vi "initialize Session Data.vi"(0 "Session in":refnum<class "Remote Connection Session.lvclass">, 11 "error in":errorcluster) -> (4 "Session out":refnum<class "Remote Connection Session.lvclass">, 15 "error out":errorcluster)   [LabVIEW 2012, in "REx.lvlib" / "Remote Connection Session.lvclass"]
uses:
  Remote Connection Session.lvclass
  <userlib>/_Session Fwk/Session - Root.lvclass
  Remote Connection Session.lvclass/Remote Connection Session.ctl
  Local Listener Session/Local Listener Session.lvclass
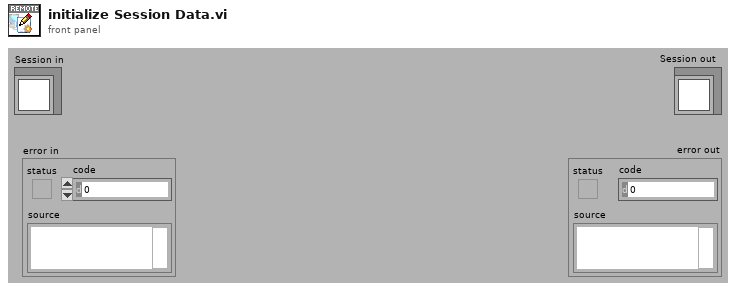
[diagram p1: front panel]
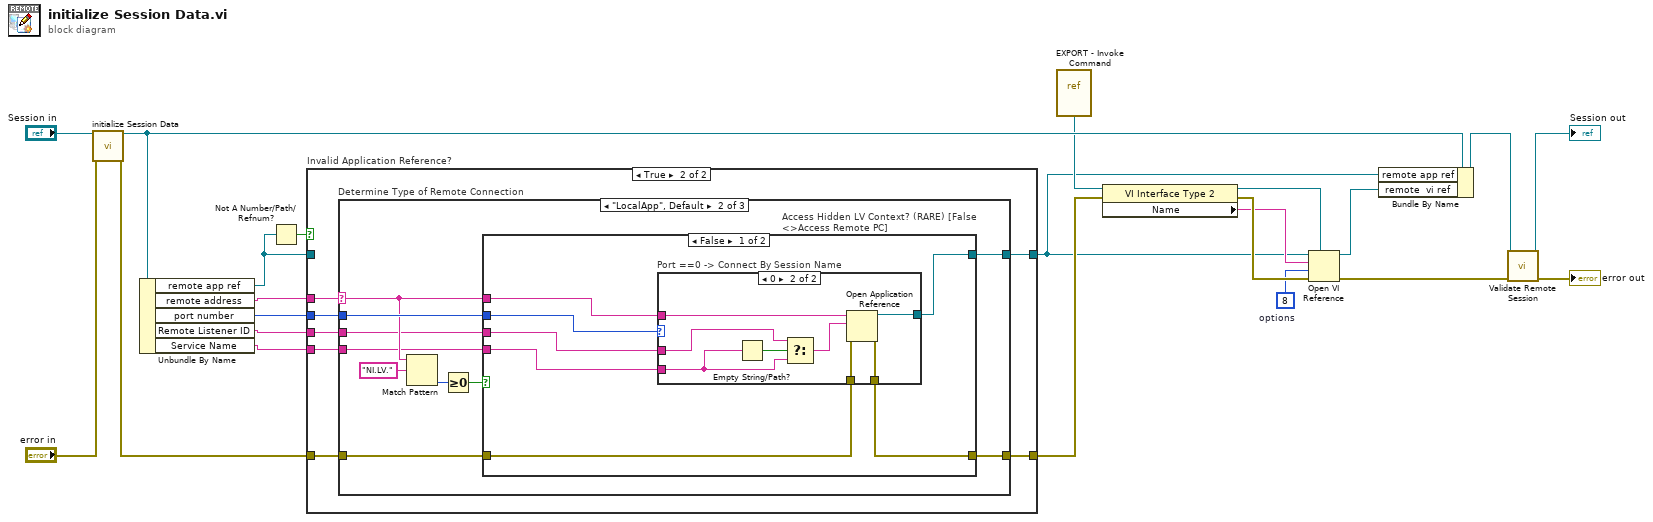
[diagram p0: block diagram]
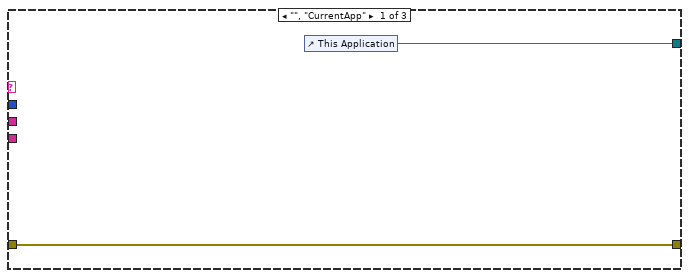
[diagram p3: hidden frame]
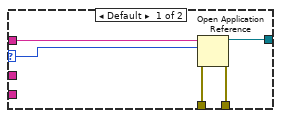
[diagram p4: hidden frame]
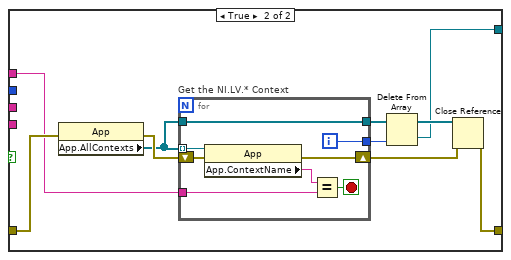
[diagram p5: hidden frame]
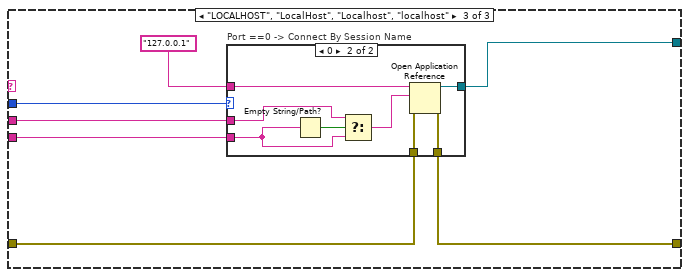
[diagram p6: hidden frame]
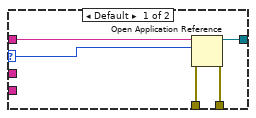
[diagram p7: hidden frame]
diagram:
  w8 = 8  # options
  n1 = call-parent "initialize Session Data.vi"("OBJ - Session in"="Session in", "error in"="error in") -> ("OBJ - Session out"=w12:refnum<class "Remote Connection Session.lvclass">, "error out"=w15:errorcluster)  [unwired: 12 in]
  n2 = Unbundle By Name(w12) -> ("remote app ref"=w18:refnum<vi>, "remote address"=w17:string, "port number"=w16:u16, "Remote Listener ID"=w5:string, "Service Name"=w6:string)
  n3 = Not A Number/Path/Refnum?(number/path/refnum=w18) -> (NaN/Path/Refnum?=w14:bool)
  n4 = case "Invalid Application Reference?" shown="True" w14 {
    tunnel: w16 -> [_ w31]
    tunnel: w15 -> [w23 w30]
    tunnel: [w23 w29] -> w9
    tunnel: w17 -> [_ w28]
    tunnel: [w24 w27] -> w3
    tunnel: w18 -> [w24 _]
    tunnel: w5 -> [_ w26]
    tunnel: w6 -> [_ w25]
    frame False {
    }
    frame True {
      n5 = case "Determine Type of Remote Connection" shown="\"LocalApp\", Default" w28 {
        selector: w28 -> [_ w37 _]
        tunnel: [w32 w43 w88] -> w27
        tunnel: [w33 w41 w87] -> w29
        tunnel: w30 -> [w33 w40 w85]
        tunnel: w31 -> [_ w42 w83]
        tunnel: w26 -> [_ w35 w84]
        tunnel: w25 -> [_ w34 w82]
        frame "", "CurrentApp" {
          n6 = control-ref of="This Application"() -> (w32:refnum<vi>)
        }
        frame "LocalApp", Default {
          n7 = Match Pattern(string=w37, regular expression="NI.LV.") -> (offset past match=w39:i32)  [unwired: 4 out]
          n8 = Greater Or Equal To 0?(x=w39) -> (x >= 0?=w36:bool)
          n9 = case "Access Hidden LV Context? (RARE) [False <>Access Remote PC]" shown="False" w36 {
            tunnel: [w47 w67] -> w43
            tunnel: w37 -> [w46 w70]
            tunnel: w42 -> [w50 _]
            tunnel: [w48 w65] -> w41
            tunnel: w40 -> [w49 w72]
            tunnel: w35 -> [w45 _]
            tunnel: w34 -> [w44 _]
            frame False {
              n10 = case "Port ==0 -> Connect By Session Name" shown="0" w50 {
                selector: w50 -> [w52 _]
                tunnel: [w55 w63] -> w47
                tunnel: [w54 w62] -> w48
                tunnel: w49 -> [w53 w61]
                tunnel: w46 -> [w51 w60]
                tunnel: w45 -> [_ w57]
                tunnel: w44 -> [_ w58]
                frame Default {
                  n11 = Open Application Reference(8:w53, 10:w52, 11:w51) -> (0:w54:errorcluster, 3:w55:refnum<vi>)  [unwired: 1 out]
                }
                frame 0 {
                  n12 = Empty String/Path?(string/path=w58) -> (empty?=w59:bool)
                  n13 = Select(t=w57, s=w59, f=w58) -> (s? t:f=w56:string)
                  n14 = Open Application Reference(8:w61, 10:w56, 11:w60) -> (0:w62:errorcluster, 3:w63:refnum<vi>)  [unwired: 1 out]
                }
              }
            }
            frame True {
              n15 = property class="App"(error in=w72) -> (error out=w73:errorcluster, "App.AllContexts"=w71:refnum<vi>[])  [unwired: 1 in, 1 out]
              n16 = for "Get the NI.LV.* Context" {
                tunnel: w71 -> [w81] mode=indexing
                shift-right: [w77] -> w64
                shift-left: w73 -> [w78]
                tunnel: w70 -> [w76]
                tunnel: [w75] -> w68
                tunnel: w71 -> [w75]
                tunnel: [w74] -> w66
                i -> [w74]
                stop <- w79 stop-if-true
                n17 = property class="App"(reference=w81, error in=w78) -> (error out=w77:errorcluster, "App.ContextName"=w80:string)  [unwired: 1 out]
                n18 = Equal?(x=w80, y=w76) -> (x = y?=w79:bool)
              }
              n19 = Delete From Array(array=w68, index=w66) -> (deleted portion=w67:refnum<vi>, array with subset deleted=w69:refnum<vi>[])  [unwired: 1 in]
              n20 = Close Reference(reference=w69, error in (no error)=w64) -> (error out=w65:errorcluster)
            }
          }
        }
        frame "LOCALHOST", "LocalHost", "Localhost", "localhost" {
          n21 = case "Port ==0 -> Connect By Session Name" shown="0" w83 {
            selector: w83 -> [w89 _]
            tunnel: [w93 w101] -> w88
            tunnel: [w92 w100] -> w87
            tunnel: "127.0.0.1" ("machine name (Local:\"\")") -> [w91 w99]
            tunnel: w85 -> [w90 w98]
            tunnel: w84 -> [_ w95]
            tunnel: w82 -> [_ w94]
            frame Default {
              n22 = Open Application Reference(8:w90, 10:w89, 11:w91) -> (0:w92:errorcluster, 3:w93:refnum<vi>)  [unwired: 1 out]
            }
            frame 0 {
              n23 = Empty String/Path?(string/path=w94) -> (empty?=w97:bool)
              n24 = Select(t=w95, s=w97, f=w94) -> (s? t:f=w96:string)
              n25 = Open Application Reference(8:w98, 10:w96, 11:w99) -> (0:w100:errorcluster, 3:w101:refnum<vi>)  [unwired: 1 out]
            }
          }
        }
      }
    }
  }
  n26 = vi-ref "EXPORT - Invoke Command.vi"() -> (w7:refnum<vi>)
  n27 = property class="VI Interface Type 2"(reference=w7, error in=w9) -> (reference out=w13:refnum<vi>, error out=w21:errorcluster, "Name"=w11:string)
  n28 = Open VI Reference(type specifier VI Refnum (for type only)=w13, application reference (local)=w3, vi path=w11, options=w8, error in (no error)=w21) -> (vi reference=w10:refnum<vi>, error out=w22:errorcluster)  [unwired: 1 out]
  n29 = Bundle By Name(cluster=w12, "remote app ref"=w3, "remote  vi ref"=w10) -> (w2:refnum<class "Remote Connection Session.lvclass">)
  n30 = call "Validate Remote Session.vi"("Session in"=w2, "error in"=w22) -> ("Session out"=→"Session out":refnum<class "Remote Connection Session.lvclass">, "error out"=→"error out":errorcluster)  [unwired: 12 in]
